vi "Modules Support.vi"(8 "error in (no error)":errorcluster) -> (0 "error out":errorcluster)   [LabVIEW 2020]
uses:
  Logging/SAVE.lvlib
  LOG/LOG.lvlib
  ALARM/QCT ALARM.lvlib
  Report/Report.lvlib
  Timer/OPC.lvlib
  Valve Control/Valve Control.lvlib
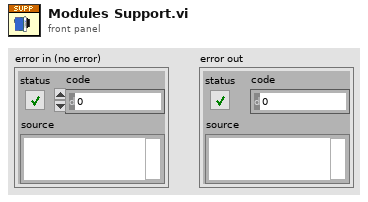
[diagram p1: front panel]
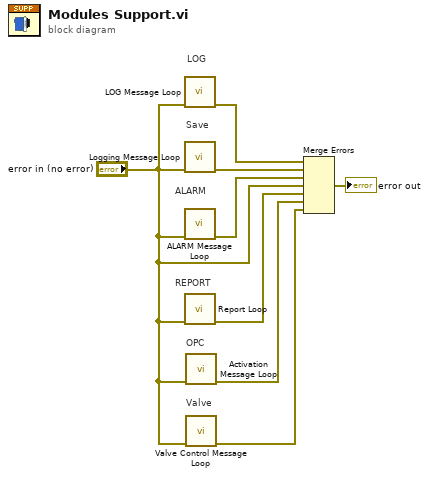
[diagram p0: block diagram]
diagram:
  # "Valve"
  # "OPC"
  # "ALARM"
  # "Save"
  # "LOG"
  # "REPORT"
  n1 = call "LOG Message Loop.vi"("error in (no error)"="error in (no error)") -> ("error out"=w6:errorcluster)  [unwired: 10 in]
  n2 = call "Logging Message Loop.vi"("error in (no error)"="error in (no error)") -> ("error out"=w8:errorcluster)  [unwired: 10 in]
  n3 = call "ALARM Message Loop.vi"("error in (no error)"="error in (no error)") -> ("error out"=w5:errorcluster)  [unwired: 10 in]
  n4 = call "Report Loop.vi"("error in (no error)"="error in (no error)") -> ("error out"=w4:errorcluster)  [unwired: 10 in]
  n5 = call "Activation Message Loop.vi"("error in (no error)"="error in (no error)") -> ("error out"=w3:errorcluster)  [unwired: 10 in]
  n6 = call "Valve Control Message Loop.vi"("error in (no error)"="error in (no error)") -> ("error out"=w2:errorcluster)  [unwired: 10 in]
  n7 = Merge Errors(w6, w8, w5, "error in (no error)", w4, w3, w2) -> (→"error out":errorcluster)
